vi "GetMaxGroup.vi"(10 "total groups":i32, 11 "key values":T1[](array[typedef])) -> (3 "Max Group":i32=3)   [LabVIEW 2017, in "McsaAnalysisLowRate.lvlib"]
uses:
  <vilib>/addons/InsightCM/Devices/Shared/Mcsa/McsaAnalysisLowRate/McsaAnalysisLowRate.lvlib
  <vilib>/addons/InsightCM/MessageBus/Base/controls/SectionKeyValues.ctl
  <vilib>/addons/InsightCM/MessageBus/Base/controls/KeyValuePair.ctl
  <vilib>/addons/InsightCM/Utilities/PropertyHelpers/PropertyHelpers.lvlib
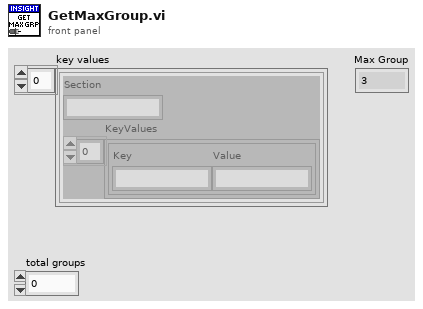
[diagram p1: front panel]
types:
  T1 = typedef "SectionKeyValues.ctl" = cluster{"Section":string, "KeyValues":T2[]}
  T2 = typedef "KeyValuePair.ctl" = cluster{"Key":string, "Value":string}
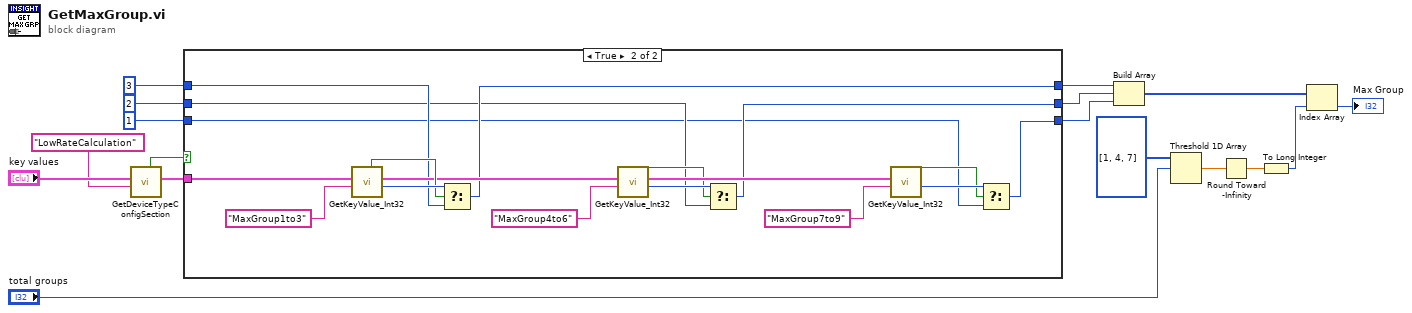
[diagram p0: block diagram]
diagram:
  n1 = call <vilib>:"GetDeviceTypeConfigSection.vi"("key"="LowRateCalculation", "key values"="key values") -> ("key value pairs out"=w9:T2[], "found"=w10:bool)  [unwired: 8 in]
  n2 = case shown="True" w10 {
    tunnel: [w18 w27] -> w17
    tunnel: [w19 w26] -> w16
    tunnel: [w20 w25] -> w15
    tunnel: w9 -> [_ w24]
    tunnel: 3 ("f") -> [w20 w23]
    tunnel: 2 ("f") -> [w19 w22]
    tunnel: 1 ("f") -> [w18 w21]
    frame False {
    }
    frame True {
      n3 = call <vilib>:"GetKeyValue_Int32.vi"("key"="MaxGroup1to3", "key value pairs"=w24) -> ("value"=w37:i32, "key value pairs out"=w33:T2[], "found"=w36:bool)  [unwired: 7 in]
      n4 = Select(t=w37, s=w36, f=w23) -> (s? t:f=w25:i32)
      n5 = call <vilib>:"GetKeyValue_Int32.vi"("key"="MaxGroup4to6", "key value pairs"=w33) -> ("value"=w35:i32, "key value pairs out"=w30:T2[], "found"=w29:bool)  [unwired: 7 in]
      n6 = Select(t=w35, s=w29, f=w22) -> (s? t:f=w26:i32)
      n7 = call <vilib>:"GetKeyValue_Int32.vi"("key"="MaxGroup7to9", "key value pairs"=w30) -> ("value"=w31:i32, "found"=w28:bool)  [unwired: 7 in, 1 out]
      n8 = Select(t=w31, s=w28, f=w21) -> (s? t:f=w27:i32)
    }
  }
  n9 = Build Array(w15, w16, w17) -> (w4:i32[])
  n10 = Threshold 1D Array(2:"total groups", 3:i32[] [1, 4, 7]) -> (0:w13:dbl)  [unwired: 1 in]
  n11 = Round Toward -Infinity(1:w13) -> (0:w12:dbl)
  n12 = To Long Integer(number=w12) -> (32bit integer=w3:i32)
  n13 = Index Array(array=w4, index=w3) -> (element=→"Max Group":i32)
